vi "Main_Console.vi"(0 "Text_File_Path":path, 5 "Sort":bool, 7 "CSV_File_Path":path, 9 "Save":bool) -> (4 "Table":string[][](table))   [LabVIEW 2021]
doc: "This VI is MainVI that Interact with user"
uses:
  Library/File_Handler_Library.lvlib
  Library/Library_Controls/Order.ctl
  Library/Library_Controls/Mode.ctl
panel:
  in  "Error_In":errorcluster
  out "Error_Out":errorcluster
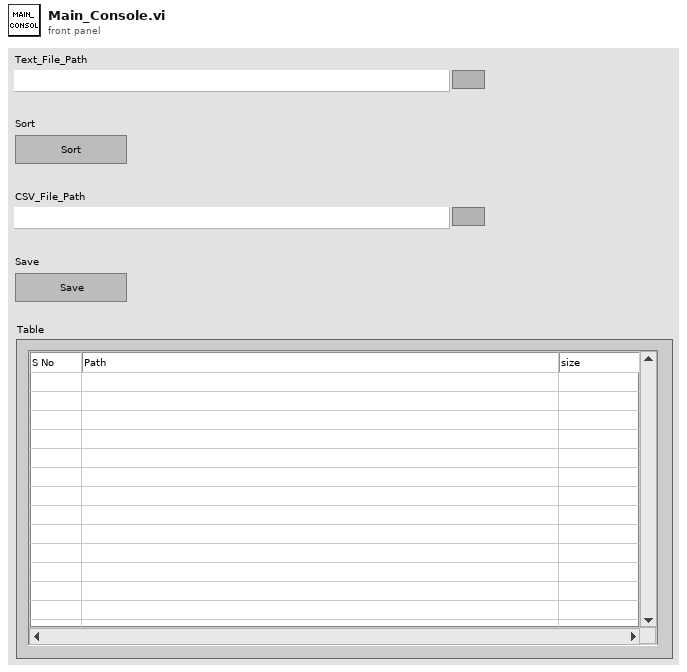
[diagram p1: front panel]
types:
  T1 = enum8{"Enabled", "Disabled", "Disabled and Grayed Out"}
  T2 = typedef "File_Handler_Library.lvlib/Mode.ctl" = enum16{"Write", "Read"}
  T3 = typedef "File_Handler_Library.lvlib/Order.ctl" = enum16{"Z to A", "A to Z"}
  T4 = enum16{"Left Button", "Center Button", "Right Button", "Window Close"}
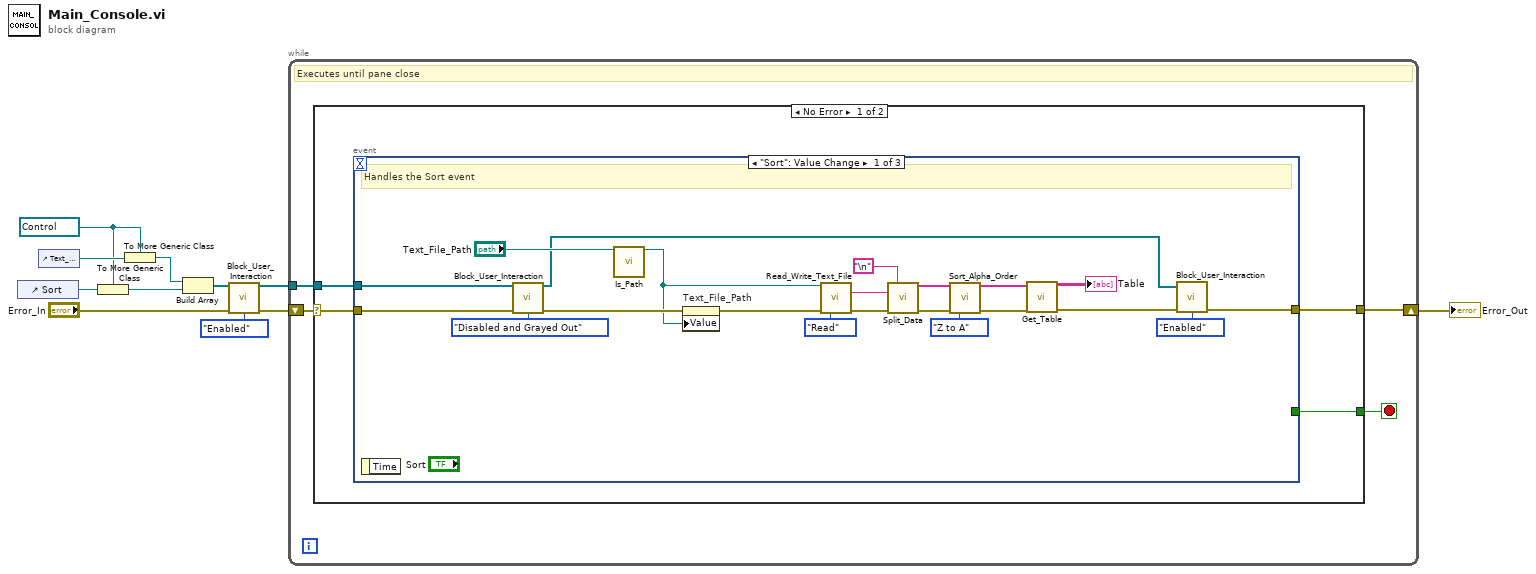
[diagram p0: block diagram]
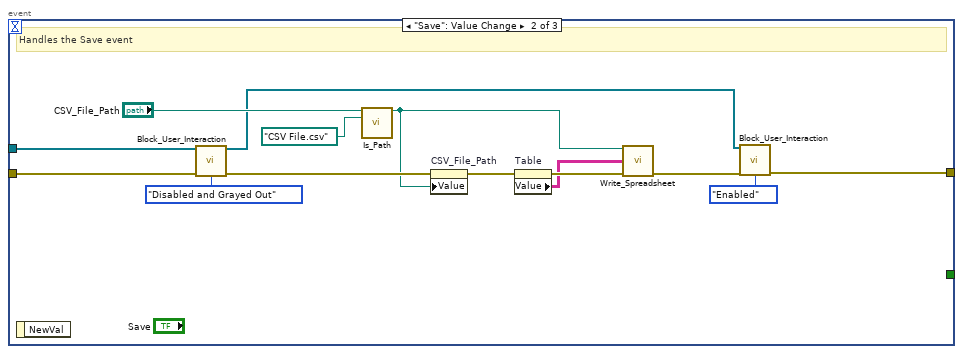
[diagram p2: hidden frame]
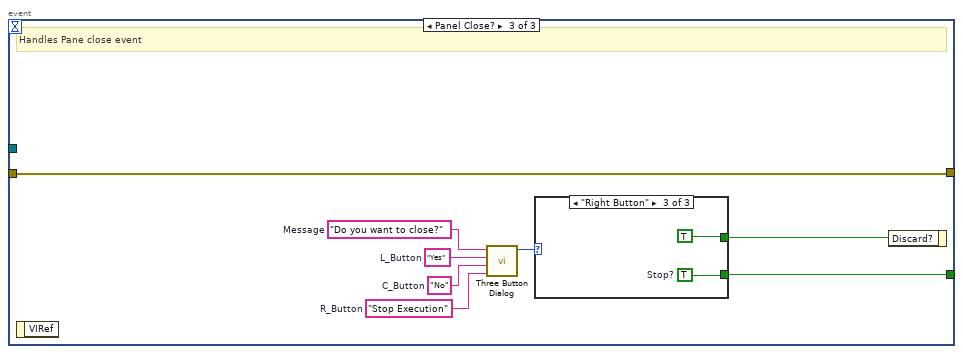
[diagram p3: hidden frame]
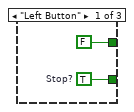
[diagram p4: hidden frame]
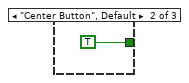
[diagram p5: hidden frame]
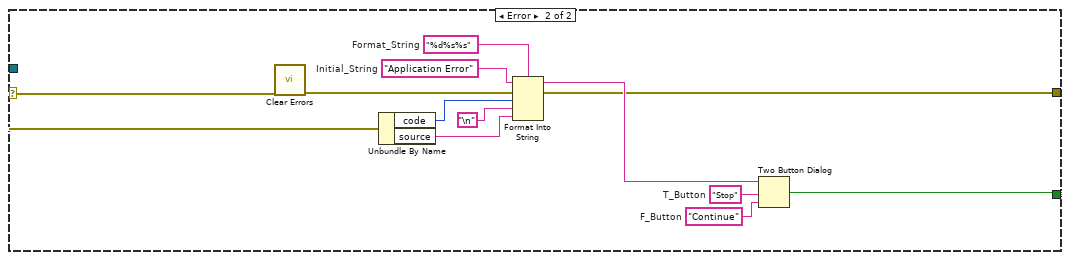
[diagram p6: hidden frame]
diagram:
  w3 = refnum<vi> refnum ("Reference_In")
  n1 = control-ref of="Sort"() -> (w6:refnum<vi>)
  n2 = control-ref of="Text_File_Path"() -> (w7:refnum<vi>)
  n3 = To More Generic Class(target class=w3, reference=w6) -> (generic class reference=w5:refnum<vi>)
  n4 = To More Generic Class(target class=w3, reference=w7) -> (generic class reference=w4:refnum<vi>)
  n5 = Build Array(w4, w5) -> (w2:refnum<vi>[])
  n6 = call "Block_User_Interaction.vi"("Reference_In"=w2, "Error_In"="Error_In", "Disabled"=T1."Enabled") -> ("Reference_Out"=w1:refnum<vi>[], "Error_Out"=w9:errorcluster)  [unwired: 11 in]
  n7 = while {
    shift-right: [w14] -> w11
    shift-left: w9 -> [w15]
    tunnel: w1 -> [w12]
    stop <- w13 stop-if-true
    # "Executes until pane close"
    n8 = case shown="No Error" w15 {
      selector: w15 -> [w19 w70]
      tunnel: [w18 w69] -> w14
      tunnel: [w17 w68] -> w13
      tunnel: w12 -> [w16 _]
      frame No Error {
        n9 = event shown="[0] \"Sort\": Value Change" {
          selector: _ -> [_ _ _]
          dyn-events: _ -> [_ _ _]
          timeout: _ -> [_ _ _]
          tunnel: w19 -> [w30 w54 w55]
          tunnel: [w22 w45 w55] -> w18
          tunnel: [_ _ w56] -> w17
          tunnel: w16 -> [w28 w50 _]
          event "Sort": Value Change {
            # "Handles the Sort event"
            n10 = event-data() -> ()  [unwired: 1 in, 1 out]
            n11 = call "Block_User_Interaction.vi"("Reference_In"=w28, "Error_In"=w30, "Disabled"=T1."Disabled and Grayed Out") -> ("Reference_Out"=w21:refnum<vi>[], "Error_Out"=w29:errorcluster)  [unwired: 11 in]
            n12 = call "Is_Path.vi"("File_Path_In"="Text_File_Path") -> ("File_Path_Out"=w26:path)  [unwired: 14 in]
            n13 = property on="Text_File_Path" class="Path"(error in=w29, "Value"=w26) -> (error out=w31:errorcluster)  [unwired: 1 in, 1 out]
            n14 = call "Read_Write_Text_File.vi"("File_Path_In"=w26, "Error_In"=w31, "Mode"=Mode."Read") -> ("Data_Out"=w38:string, "Error_Out"=w40:errorcluster)  [unwired: 10 in, 1 out]
            n15 = call "Split_Data.vi"("Delimiter"="\n", "Data_In"=w38, "Error_In"=w40) -> ("Split_Data_Out"=w36:string[], "Error_Out"=w39:errorcluster)  [unwired: 11 in]
            n16 = call "Sort_Alpha_Order.vi"("Split_Data"=w36, "Error_In"=w39, "Order (Z to A)"=Order."Z to A") -> ("Sorted_Array"=w34:string[], "Error_Out"=w32:errorcluster)  [unwired: 11 in]
            n17 = call "Get_Table.vi"("Sorted_Array"=w34, "Error_In"=w32) -> ("Table"=→"Table":string[][], "Error_Out"=w23:errorcluster)  [unwired: 12 in]
            n18 = call "Block_User_Interaction.vi"("Reference_In"=w21, "Error_In"=w23, "Disabled"=T1."Enabled") -> ("Error_Out"=w22:errorcluster)  [unwired: 11 in, 1 out]
          }
          event "Save": Value Change {
            # "Handles the Save event"
            n19 = event-data() -> ()  [unwired: 1 in, 1 out]
            n20 = call "Block_User_Interaction.vi"("Reference_In"=w50, "Error_In"=w54, "Disabled"=T1."Disabled and Grayed Out") -> ("Reference_Out"=w44:refnum<vi>[], "Error_Out"=w49:errorcluster)  [unwired: 11 in]
            n21 = call "Is_Path.vi"("File_Path_In"="CSV_File_Path", "File_Name"=path "CSV File.csv") -> ("File_Path_Out"=w47:path)  [unwired: 13 in]
            n22 = property on="CSV_File_Path" class="Path"(error in=w49, "Value"=w47) -> (error out=w48:errorcluster)  [unwired: 1 in, 1 out]
            n23 = property on="Table" class="Tbl (strict)"(error in=w48) -> (error out=w52:errorcluster, "Value"=w51:string[][])  [unwired: 1 in, 1 out]
            n24 = call "Write_Spreadsheet.vi"("File_Path_In"=w47, "Table"=w51, "Error_In"=w52) -> ("Error_Out"=w46:errorcluster)  [unwired: 11 in, 1 out]
            n25 = call "Block_User_Interaction.vi"("Reference_In"=w44, "Error_In"=w46, "Disabled"=T1."Enabled") -> ("Error_Out"=w45:errorcluster)  [unwired: 11 in, 1 out]
          }
          event Panel Close? {
            w59 = "Stop Execution"  # R_Button
            w60 = "No"  # C_Button
            w61 = "Yes"  # L_Button
            w62 = "Do you want to close?"  # Message
            # "Handles Pane close event"
            n26 = event-data() -> ()  [unwired: 1 in, 1 out]
            n27 = call <vilib>:"Three Button Dialog.vi"("Right Button Text (\"Cancel\")"=w59, "Center Button Text (\"No\")"=w60, "Left Button Text (\"Yes\")"=w61, "message"=w62) -> ("Which Button?"=w58:T4)  [unwired: 7 in]
            n28 = case shown="\"Right Button\"" w58 {
              tunnel: [FALSE TRUE TRUE] -> w57
              tunnel: [w63 _ w67] -> w56
              frame "Left Button" {
                w63 = TRUE  # Stop?
              }
              frame "Center Button", Default {
              }
              frame "Right Button" {
                w67 = TRUE  # Stop?
              }
            }
            n29 = event-data("Discard?"=w57) -> ()  [unwired: 1 in, 1 out]
          }
        }
      }
      frame Error {
        w75 = "%d%s%s"  # Format_String
        w76 = "Application Error"  # Initial_String
        w77 = "Stop"  # T_Button
        w78 = "Continue"  # F_Button
        n30 = call <vilib>:"Clear Errors.vi"("error in (no error)"=w70) -> ("error out"=w73:errorcluster)  [unwired: 5 in, 1 out]
        n31 = Unbundle By Name(w70) -> ("code"=w72:i32, "source"=w71:string)
        n32 = Format Into String(format string=w75, initial string=w76, error in=w73, w72, "\n", w71) -> (resulting string=w79:string, error out=w69:errorcluster)
        n33 = Two Button Dialog(message=w79, 1:w78, 2:w77) -> (T button?=w68:bool)
      }
    }
  }
  "Error_Out" <- w11
